vi "Prepare Source.vi"(0 "instrument handle":refnum<k15>, 7 "Initial Voltage Level (V)":dbl, 11 "error in (no error)":errorcluster) -> (15 "error out":errorcluster)   [LabVIEW 2020]
uses:
  <instrlib>/niDCPower/nidcpower.llb/niDCPower Source Mode.ctl
  <instrlib>/niDCPower/nidcpower.llb/niDCPower Output Function.ctl
  <instrlib>/niDCPower/nidcpower.llb/niDCPower Wait For Event - Event.ctl
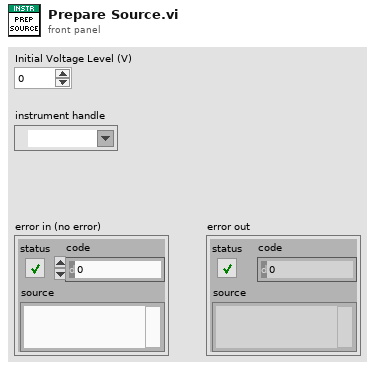
[diagram p1: front panel]
types:
  T1 = typedef "niDCPower Wait For Event - Event.ctl" = i32
  T2 = typedef "niDCPower Output Function.ctl" = i32
  T3 = typedef "niDCPower Source Mode.ctl" = i32
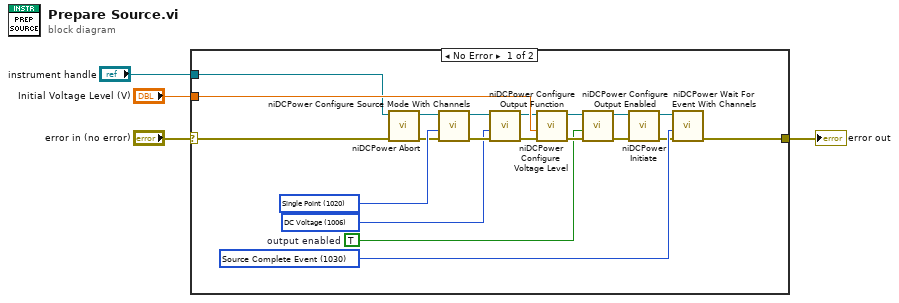
[diagram p0: block diagram]
diagram:
  n1 = case shown="No Error" "error in (no error)" {
    selector: "error in (no error)" -> [w19 w25]
    tunnel: "Initial Voltage Level (V)" -> [w24 _]
    tunnel: [w22 w25] -> w3
    tunnel: "instrument handle" -> [w5 _]
    frame No Error {
      w23 = T1 1030 items=["Source Complete Event"=1030, "Measure Complete Event"=1031, "Sequence Iteration Complete Event"=1032, "Sequence Engine Done Event"=1033, "Pulse Complete Event"=1051, "Ready For Pulse Trigger Event"=1052] ("event")
      w14 = TRUE  # output enabled
      w8 = T2 1006 items=["DC Voltage"=1006, "DC Current"=1007, "Pulse Voltage"=1049, "Pulse Current"=1050] ("output function")
      w11 = T3 1020 items=["Single Point"=1020, "Sequence"=1021] ("source mode")
      n2 = call <instrlib>:"niDCPower Abort.vi"("error in (no error)"=w19, "instrument handle"=w5) -> ("error out"=w7:errorcluster, "instrument handle out"=w6:refnum<k15>)  [unwired: 8 in]
      n3 = call <instrlib>:"niDCPower Configure Source Mode With Channels.vi"("error in (no error)"=w7, "source mode"=w11, "instrument handle"=w6) -> ("error out"=w9:errorcluster, "instrument handle out"=w10:refnum<k15>)  [unwired: 7 in]
      n4 = call <instrlib>:"niDCPower Configure Output Function.vi"("error in (no error)"=w9, "output function"=w8, "instrument handle"=w10) -> ("error out"=w12:errorcluster, "instrument handle out"=w13:refnum<k15>)  [unwired: 7 in]
      n5 = call <instrlib>:"niDCPower Configure Voltage Level.vi"("error in (no error)"=w12, "voltage level"=w24, "instrument handle"=w13) -> ("error out"=w15:errorcluster, "instrument handle out"=w18:refnum<k15>)  [unwired: 7 in]
      n6 = call <instrlib>:"niDCPower Configure Output Enabled.vi"("error in (no error)"=w15, "output enabled"=w14, "instrument handle"=w18) -> ("error out"=w16:errorcluster, "instrument handle out"=w17:refnum<k15>)  [unwired: 7 in]
      n7 = call <instrlib>:"niDCPower Initiate.vi"("error in (no error)"=w16, "instrument handle"=w17) -> ("error out"=w20:errorcluster, "instrument handle out"=w21:refnum<k15>)  [unwired: 8 in]
      n8 = call <instrlib>:"niDCPower Wait For Event With Channels.vi"("error in (no error)"=w20, "event"=w23, "instrument handle"=w21) -> ("error out"=w22:errorcluster)  [unwired: 7 in, 1 out]
    }
    frame Error {
    }
  }
  "error out" <- w3
